vi "FTW-Test-Actor-Core_Initialize.vi"(0 "Initialization Sequence":string, 5 "FTW Actor Instance Configuration":string, 11 "error in (no error)":errorcluster) -> (4 "Actor Template-Core out":refnum<class "FTW-Test-Actor-Core.lvclass">, 6 "Event Refnums":T1, 10 "Refresh Period":dbl, 15 "error out":errorcluster)   [LabVIEW 2018, in "FTW-Test-Actor-Core.lvclass"]
uses:
  FTW-Test-Actor-Core.lvclass
  source/actor/Message/Request/FTW-Message-IncomingRequest.lvclass
  source/actor/Message/Base/FTW-Message.lvclass
  FTW-Test-Actor-Core.lvclass/FTW-Test-Actor-Core.ctl
  a0ab2543-1c37-4a69-881f-c8e8dbee0ff8.vi
  source/JSON/core/FTW-JSON-Core-EncodingFlags.vi
  source/Reflection/FTW-Reflection-Type.vi
  source/JSON/FTW-JSON-Parse.vi
  source/container/FTW-Container-GetFlattenedValue.vi
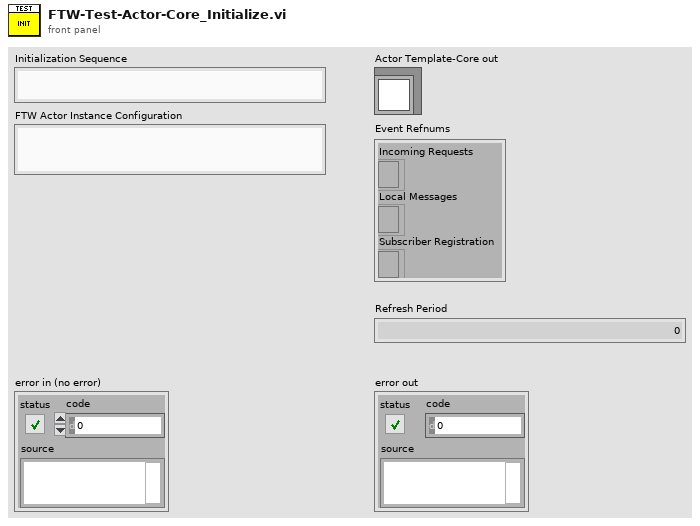
[diagram p1: front panel]
types:
  T1 = cluster{"Incoming Requests":refnum<event-registration>, "Local Messages":refnum<event-registration>, "Subscriber Registration":refnum<event-registration>}
  T2 = cluster{"My Data":bool, "Refresh Period":dbl, "Fail Initialization":bool}
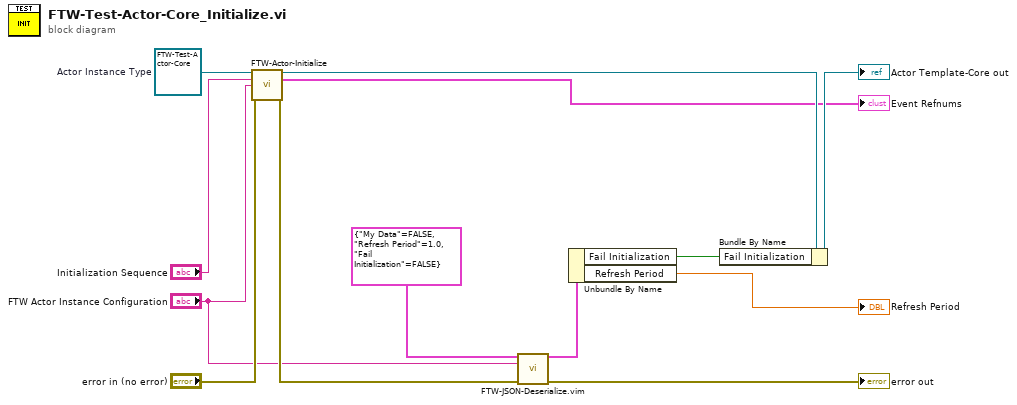
[diagram p0: block diagram]
diagram:
  w13 = refnum<class "FTW-Test-Actor-Core.lvclass"> refnum  # Actor Instance Type
  n1 = call-dynamic "FTW-Actor-Initialize.vi"("FTW Actor Instance Type"=w13, "Initialization Job Sequence"="Initialization Sequence", "Actor Instance Configuration"="FTW Actor Instance Configuration", "error in"="error in (no error)") -> ("FTW Actor Instance"=w7:refnum<class "FTW-Test-Actor-Core.lvclass">, "Event Refnums"=→"Event Refnums":T1, "error out"=w5:errorcluster)  [unwired: 9 in]
  n2 = call "FTW-JSON-Deserialize.vim"("Type In"=T2 {"My Data"=FALSE, "Refresh Period"=1.0, "Fail Initialization"=FALSE} ("Type and Defaults"), "JSON String"="FTW Actor Instance Configuration", "error in"=w5) -> ("Type Out"=w9:T2, "error out"=→"error out":errorcluster)  [unwired: 11 in]
  n3 = Unbundle By Name(w9) -> ("Fail Initialization"=w8:bool, "Refresh Period"=→"Refresh Period":dbl)
  n4 = Bundle By Name(cluster=w7, "Fail Initialization"=w8) -> (→"Actor Template-Core out":refnum<class "FTW-Test-Actor-Core.lvclass">)
